vi "Test IPS120 comms.vi"(8 "Error In":errorcluster, 9 "Command 2":string="J1.5\r", 10 "Command 1":string="A1\r", 11 "VISA resource name":refnum<visa-resource-name>) -> (0 "Error Out":errorcluster, 3 "VISA resource name out":refnum<visa-resource-name>)   [LabVIEW 2018]
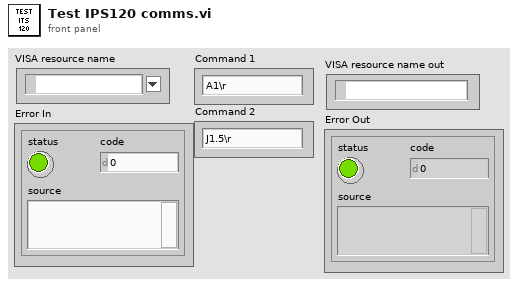
[diagram p1: front panel]
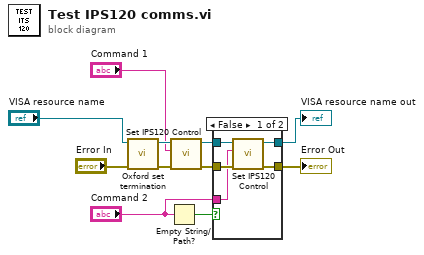
[diagram p0: block diagram]
diagram:
  n1 = call "Oxford set termination.vi"("error in (no error)"="Error In", "VISA resource name"="VISA resource name") -> ("error out"=w11:errorcluster, "VISA resource name out"=w9:refnum<visa-resource-name>)  [unwired: 8 in]
  n2 = Empty String/Path?(string/path="Command 2") -> (empty?=w1:bool)
  n3 = call "Set IPS120 Control.vi"("Error In"=w11, "Command string"="Command 1", "VISA resource name"=w9) -> ("Error Out"=w6:errorcluster, "VISA resource name out"=w5:refnum<visa-resource-name>)  [unwired: 7 in]
  n4 = case shown="False" w1 {
    tunnel: w6 -> [w16 w17]
    tunnel: w5 -> [w15 w18]
    tunnel: [w14 w18] -> w4
    tunnel: "Command 2" -> [w13 _]
    tunnel: [w12 w17] -> w3
    frame False {
      n5 = call "Set IPS120 Control.vi"("Error In"=w16, "Command string"=w13, "VISA resource name"=w15) -> ("Error Out"=w12:errorcluster, "VISA resource name out"=w14:refnum<visa-resource-name>)  [unwired: 7 in]
    }
    frame True {
    }
  }
  "VISA resource name out" <- w4
  "Error Out" <- w3
